vi "Read Setpoints.vi"(8 "error in (no error)":errorcluster, 11 "Owlstone GEN-SYS in":refnum<class "Owlstone GEN-SYS.lvclass">) -> (0 "error out":errorcluster, 2 "Setpoints":T1={"OVG-4"={"Oven Temperature"=25, "Sample Flow Rate"=50, "Split Flow Status"=0, "Split Flow Rate"=50}, "OHG-4"={"Wet Air Flow"=0}} {"OHG-4"."Wet Air Flow" min=300 max=3000 scale=300.0..3000.0; "OVG-4"."Split Flow Status" items=["Closed", "Open"]; "OVG-4"."Split Flow Rate" min=300 max=3000 scale=50.0..3000.0; "OVG-4"."Sample Flow Rate" min=50 max=500 scale=50.0..500.0; "OVG-4"."Oven Temperature" min=25 max=100 scale=25.0..100.0}, 3 "Owlstone GEN-SYS out":refnum<class "Owlstone GEN-SYS.lvclass">)   [LabVIEW 2011, in "Owlstone GEN-SYS.lvclass"]
uses:
  Owlstone GEN-SYS.lvclass
  Gen-Sys Setpoints.ctl
  Owlstone GEN-SYS.lvclass/Owlstone GEN-SYS.ctl
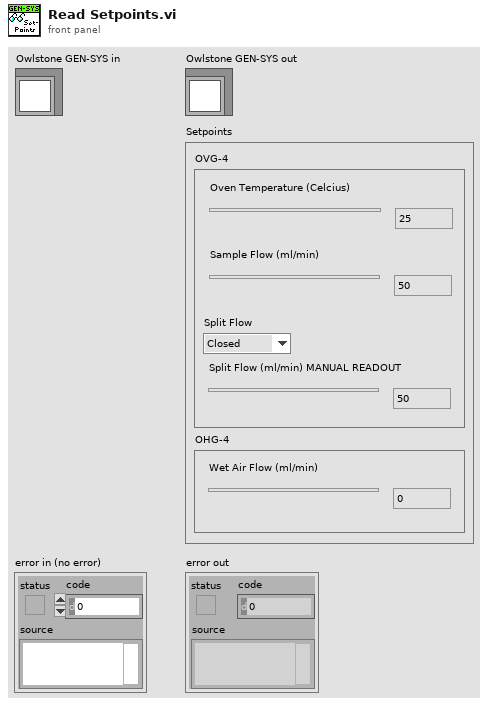
[diagram p1: front panel]
types:
  T1 = typedef "Owlstone GEN-SYS.lvclass/Gen-Sys Setpoints.ctl" = cluster{"OVG-4":cluster{"Oven Temperature":i32, "Sample Flow Rate":i32, "Split Flow Status":u16, "Split Flow Rate":i32}, "OHG-4":cluster{"Wet Air Flow":i32}}
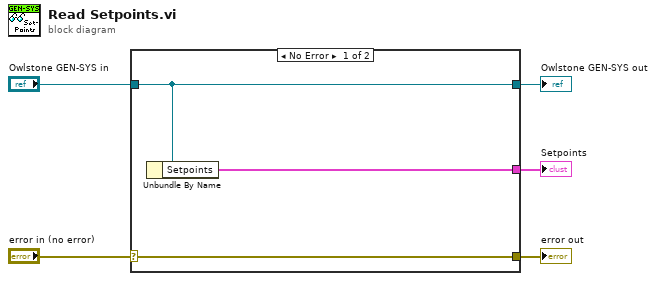
[diagram p0: block diagram]
diagram:
  n1 = case shown="No Error" "error in (no error)" {
    selector: "error in (no error)" -> [w8 w9]
    tunnel: [w8 w9] -> w4
    tunnel: [w7 w10] -> w2
    tunnel: "Owlstone GEN-SYS in" -> [w7 w10]
    tunnel: [w6 _] -> w1
    frame No Error {
      n2 = Unbundle By Name(w7) -> ("Setpoints"=w6:T1)
    }
    frame Error {
    }
  }
  "error out" <- w4
  "Owlstone GEN-SYS out" <- w2
  "Setpoints" <- w1
